vi "myRIO_BRig_RT_dataLC_Reward_Trial_l2.vi"() -> (2 "output_Reward_Trial_l2":i32)   [LabVIEW 2014]
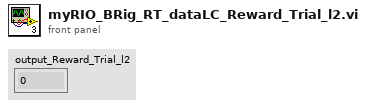
[diagram p1: front panel]
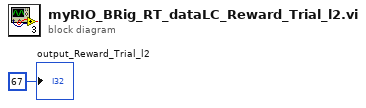
[diagram p0: block diagram]
diagram:
  "output_Reward_Trial_l2" <- 67 ("output_iBlock")
